vi "Wait.vi"() -> ()   [LabVIEW 2017]
panel:
  in  "Time":dbl
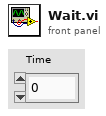
[diagram p1: front panel]
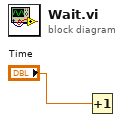
[diagram p0: block diagram]
diagram:
  n1 = Increment(x="Time") -> ()  [unwired: 1 out]
